vi "Simulation DIP.vi"() -> ()   [LabVIEW 2014]
uses:
  <vilib>/Simulation/Scripting/Companion Diagram/SimConfigNode/SimParams.ctl
  <vilib>/Simulation/Scripting/Companion Diagram/SimConfigNode/_simSolvers.ctl
  <vilib>/Simulation/Implementation/Shared/SIMSCR Execution Mode.ctl
  <vilib>/Simulation/Param Hierarchy/Typedefs/SIMPH Param Control Actions.ctl
  <vilib>/Simulation/Implementation/Shared/NILVSim_ParamChanged.vi
  <vilib>/Simulation/Implementation/Shared/NILVSIM_BeginStep.vi
  <vilib>/Simulation/Utility/Implementation/SIM Halt.vi
  <vilib>/Simulation/SignalArithmetic/Implementation/NILVSim Gain.llb/SIM Gain (scalar).vi
  <vilib>/Simulation/Implementation/Shared/SIM Is Init or Final Stage.vi
  <vilib>/Simulation/ContinuousLinear/Implementation/NILVSim State Space.llb/SIM State Space Distributor (SISO CD).vi
  <vilib>/Simulation/SignalArithmetic/Implementation/NILVSim Gain.llb/SIM Gain (vector,MatrixGain).vi
  <vilib>/Simulation/ContinuousLinear/Implementation/NILVSim State Space.llb/SIM State Space Collector (SISO CD).vi
  <vilib>/Simulation/SignalArithmetic/Implementation/NILVSim Gain.llb/SIM Gain (vector).vi
  <vilib>/Simulation/Implementation/Shared/NILVSim_Manager.vi
  <vilib>/Utility/error.llb/Clear Errors.vi
  <vilib>/Simulation/Implementation/Shared/NILVSim_FinalizeModel.vi
  <vilib>/addons/Control Design/_Model Construction/Model Creation.llb/Model Creation SubVI/cd_Create State Space Model.vi
  <vilib>/addons/Control Design/_Utility/Model Viewer.llb/Model Viewer SubVI/cd_Draw State-Space Equation (SS).vi
  <vilib>/addons/Control Design/_State Feedback Control/State Feedback Control.llb/State Feedback Control SubVis/cd_Linear Quadratic Regulator.vi
  <vilib>/Simulation/Implementation/Shared/SIM Unbundle Sim Info.vi
  <vilib>/Simulation/Implementation/Shared/NILVSim_Initialize.vi
  <vilib>/Simulation/Utility/Implementation/NILVSim Get Time and IsAcceptedStep.vi
  <vilib>/Simulation/Implementation/Shared/SIMSH Read Queue.vi
  <vilib>/Simulation/Implementation/Shared/NILVSim_GetModelError.vi
  <vilib>/Simulation/Implementation/Shared/SIM Bundle Sim Info.vi
  <vilib>/Simulation/Scripting/Companion Diagram/SimConfigNode/SimDog.xnode
  NL-Modell-Doppelpendel.vi
  <vilib>/addons/Control Design/_Model Construction/Model Typedefs.llb/CD State Space Model (MIMO).ctl
  <vilib>/addons/Control Design/_Model Construction/Model Typedefs.llb/CD General Elements.ctl
  <vilib>/Simulation/Implementation/XNodeFramework/SimXNode/SimX.xnode
  <vilib>/addons/Control Design/_Model Construction/NI_LinSys_Model Typedefs.lvlib
  <vilib>/addons/Control Design/_State Feedback Control/NI_CD_State Feedback Control.lvlib
  <vilib>/addons/Control Design/_Utility/NI_CD_Model Viewer.lvlib
  <vilib>/addons/Control Design/_Model Construction/NI_LinSys_Model Creation.lvlib
  <vilib>/Simulation/ContinuousLinear/Implementation/NILVSim State Space.llb/SIM State Space (SISO CD).vi
  <vilib>/Simulation/Implementation/Shared/NI_SIM_Implementation.lvlib
panel:
  in  "n":dbl
  out "E p 2":cluster{" 4":sgl, " 4":sgl, " 4":sgl}(graph)
  out "E p":sgl(graph)
  out "E t":dbl(graph)
  in  "ke":dbl
  in  "kv":dbl
  in  "kx":dbl
  in  "Regler 2":bool
  out "Winkel 2(Grad)":dbl(graph)=-0.008492510240475513
  out "Winkelgeschwindigkeit 2":cluster{dbl, "x4_":dbl}(graph)={5.3984229717087e-05, "x4_"=5.3984229717087e-05}
  in  "Regler":enum16{"kein", "PBR", "LQR"}(ring)=enum."LQR"
  in  "Winkelg.2_t0":dbl
  in  "Winkel2_t0 (Grad)":dbl
  in  "Winkelg.1_t0":dbl
  in  "Position_t0 (m)":dbl
  out "Kraft in N":dbl=-0.0022267318727753616
  out "Winkelgesch. Simuliert":dbl=1.2061069581493266e-05
  out "Winkel1  (rad)":dbl=-2.7704816976115154e-05
  out "Geschwindigkeit 2":dbl=0.00013263924275168403
  out "Position":dbl=0.9161585295653075
  in  "Strecke":T1(ring)
  out "State-Space Equation":picture
  out "Position (mm)":cluster{"output":dbl, "output":dbl}(graph)={"output"=100.0, "output"=0.9161585295653075}
  out "Winkel 1(Grad)":dbl(graph)=-0.001587369084913794
  out "Kraft (N)":dbl(graph)=-0.0022267318727753616
  out "Geschwindigkeit":dbl(graph)=0.00013263924275168403
  out "Winkelgeschwindigkeit 1":cluster{dbl, "x4_":dbl}(graph)={1.2061069581493266e-05, "x4_"=1.2061069581493266e-05}
  out "K":dbl[][](array[numeric])=[[99.99999999995181, -969.5856366468216, 394.3194914179953, 252.01094744906607, 27.114441675359792, 156.37982209545834]] format="%.2f"
  in  "Q":dbl[][](array[numeric])=[[100.0, 0.0, 0.0, 0.0, 0.0, 0.0], [0.0, 1.0, 0.0, 0.0, 0.0, 0.0], [0.0, 0.0, 100.0, 0.0, 0.0, 0.0], [0.0, 0.0, 0.0, 1.0, 0.0, 0.0], [0.0, 0.0, 0.0, 0.0, 1.0, 0.0], [0.0, 0.0, 0.0, 0.0, 0.0, 1.0]] format="%.2f"
  in  "R":dbl[][](array[numeric])=[[0.01]] format="%.5f"
  in  "Winkel1_t0 (Grad)":dbl
  in  "Sollwert Amplitude (mm)":dbl=100.0
  in  "Stop Button":bool
  # "Anfangswerte"
  # "PBR"
  # "LQR Regler"
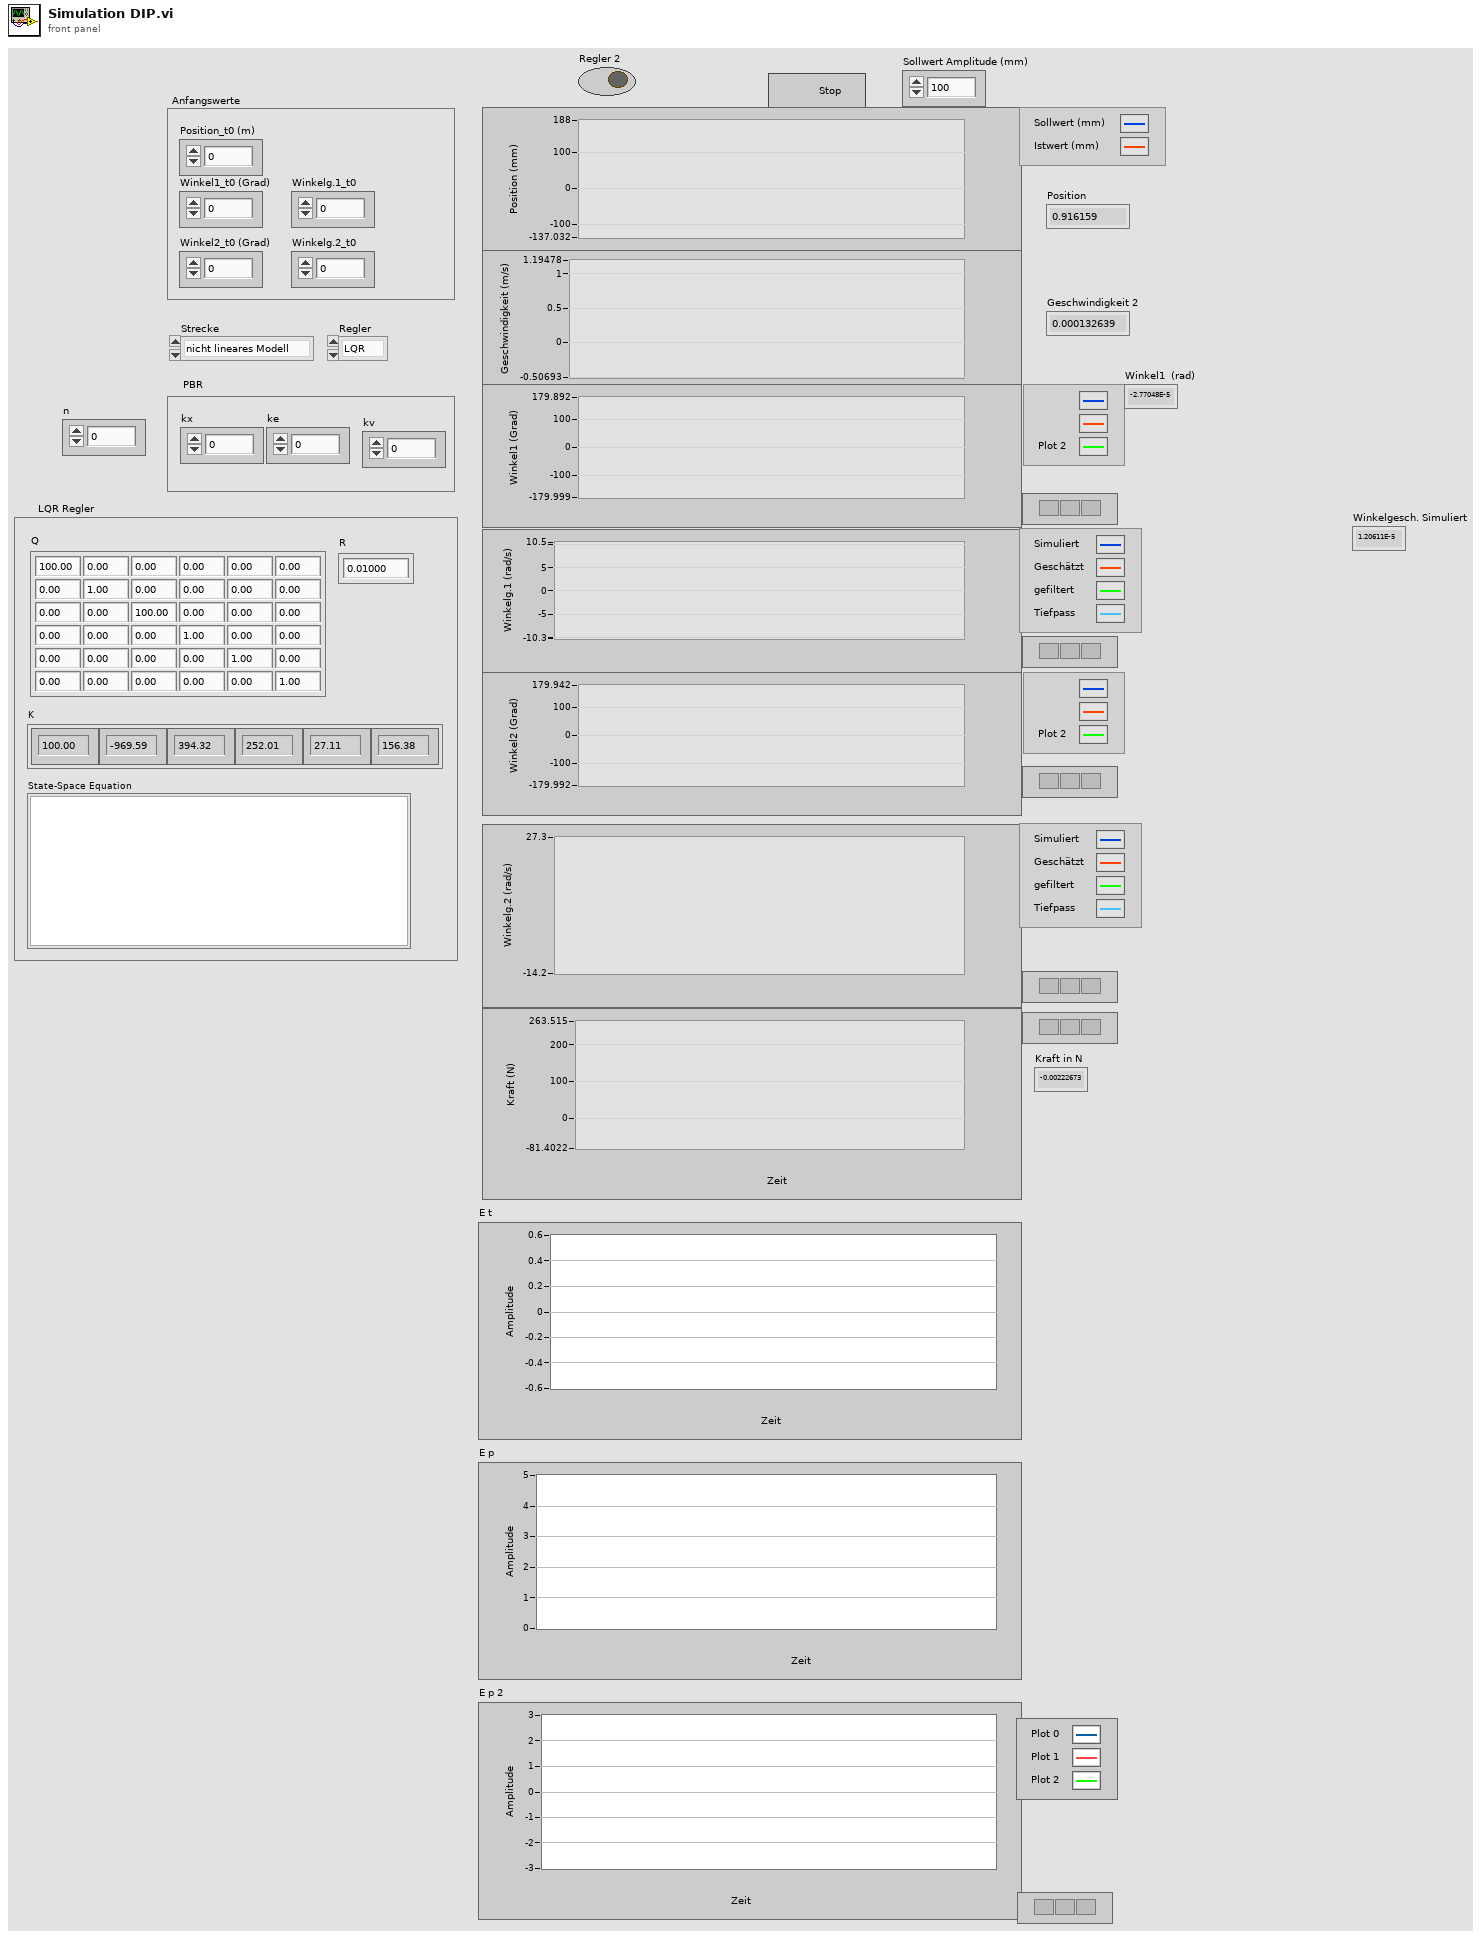
[diagram p1: front panel]
types:
  T1 = enum16{"nicht lineares Modell", "lineares Modell"}
  T2 = typedef "NI_LinSys_Model Typedefs.lvlib/CD State Space Model (MIMO).ctl" = cluster{"properties":T3, "A":dbl[][], "B":dbl[][], "C":dbl[][], "D":dbl[][], "StateNames":string[], "Transport Delay":dbl[][]}
  T3 = typedef "NI_LinSys_Model Typedefs.lvlib/CD General Elements.ctl" = cluster{"Model name":string, "Input names":string[], "Output names":string[], "Input Delays":dbl[], "Output Delays":dbl[], "Sampling Time":dbl, "Notes":string}
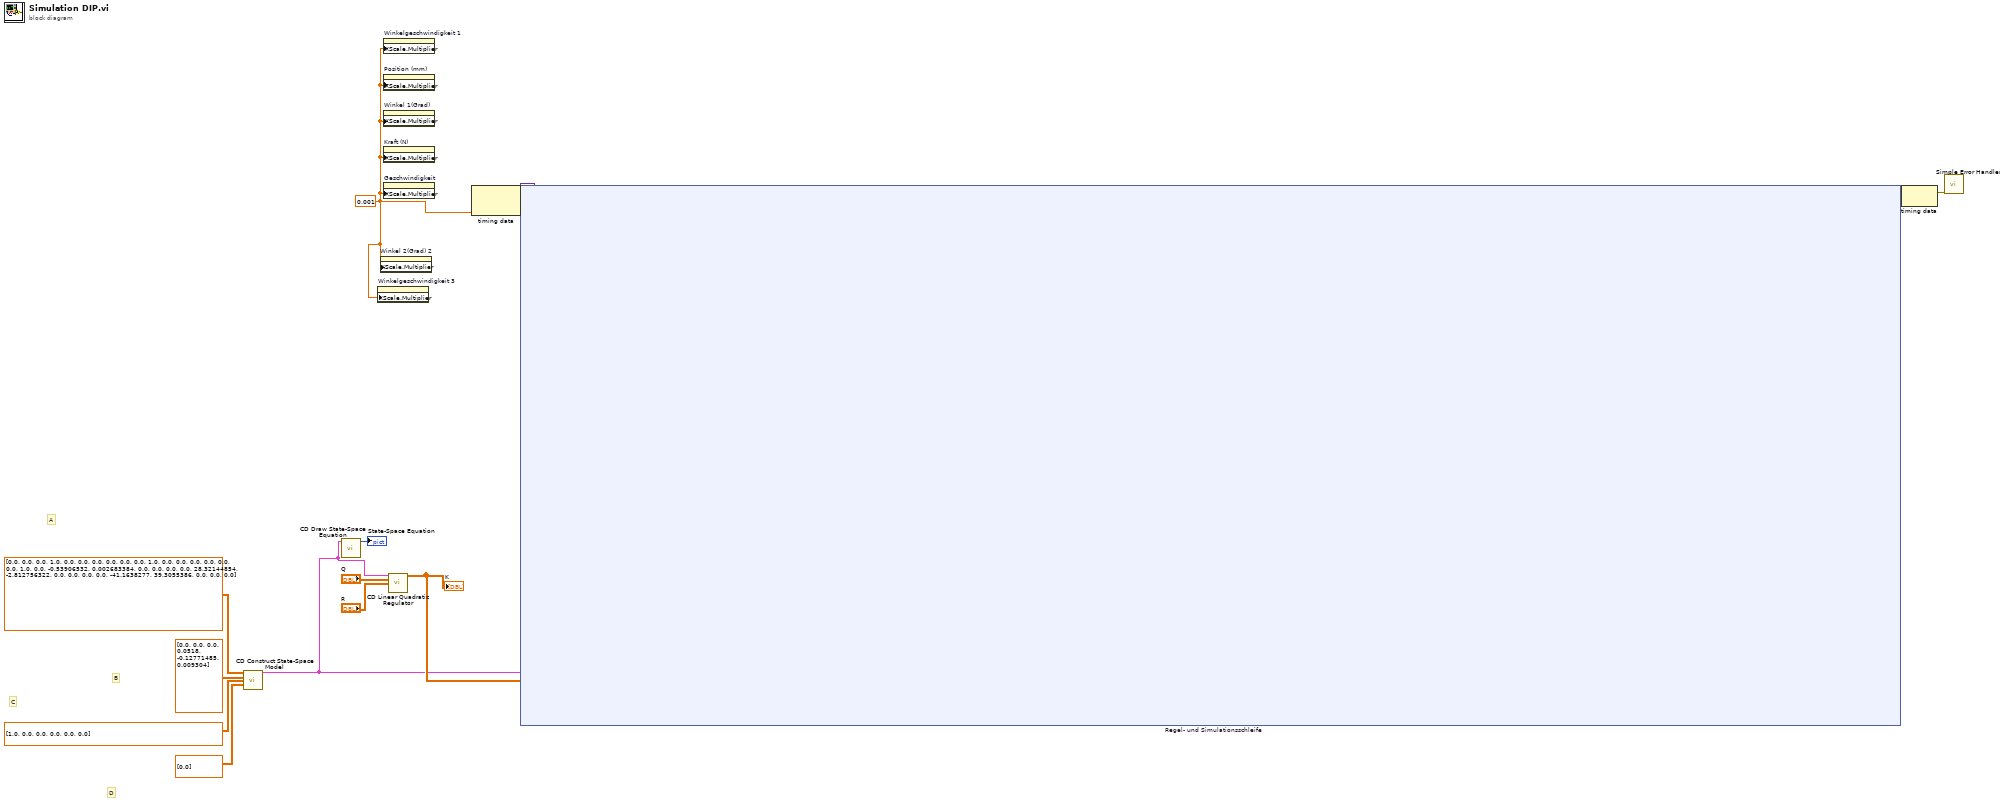
[diagram p0: block diagram]
diagram:
  w6 = 0.001 ("Step Size (s)")
  # "D"
  # "C"
  # "B"
  # "A"
  n1 = call-poly <vilib>:"CD Construct State-Space Model.vi"("A"=dbl[][] [[0.0, 0.0, 0.0, 1.0, 0.0, 0.0], [0.0, 0.0, 0.0, 0.0, 1.0, 0.0], [0.0, 0.0, 0.0, 0.0, 0.0, 1.0], [0.0, -0.53906532, 0.002683384, 0.0, 0.0, 0.0], [0.0, 28.32144854, -2.812756322, 0.0, 0.0, 0.0], [0.0, -41.1638277, 39.3055386, 0.0, 0.0, 0.0]], "B"=dbl[][] [[0.0], [0.0], [0.0], [0.0518], [-0.12771485], [0.009304]], "C"=dbl[][] [[1.0, 0.0, 0.0, 0.0, 0.0, 0.0]], "D"=dbl[][] [[0.0]]) -> ("State-Space Model"=w1:T2)  [unwired: 10 in, 1 out]
  n2 = call-poly <vilib>:"CD Draw State-Space Equation.vi"("State-Space Model"=w1) -> ("Equation"=→"State-Space Equation":picture)  [unwired: 8 in, 2 out]
  n3 = property on="Winkelgeschwindigkeit 3" class="SVDiagr (strikt)"("XScale.Multiplier"=w6) -> ()  [unwired: 2 in, 2 out]
  n4 = property on="Winkel 2(Grad) 2" class="SVDiagr (strikt)"("XScale.Multiplier"=w6) -> ()  [unwired: 2 in, 2 out]
  n5 = property on="Winkelgeschwindigkeit 1" class="SVDiagr (strikt)"("XScale.Multiplier"=w6) -> ()  [unwired: 2 in, 2 out]
  n6 = property on="Position (mm)" class="SVDiagr (strikt)"("XScale.Multiplier"=w6) -> ()  [unwired: 2 in, 2 out]
  n7 = property on="Winkel 1(Grad)" class="SVDiagr (strikt)"("XScale.Multiplier"=w6) -> ()  [unwired: 2 in, 2 out]
  n8 = property on="Kraft (N)" class="SVDiagr (strikt)"("XScale.Multiplier"=w6) -> ()  [unwired: 2 in, 2 out]
  n9 = property on="Geschwindigkeit" class="SVDiagr (strikt)"("XScale.Multiplier"=w6) -> ()  [unwired: 2 in, 2 out]
  n10 = call-poly <vilib>:"CD Linear Quadratic Regulator.vi"("State-Space Model"=w1, "Q"="Q", "R"="R") -> ("Optimal Gain (K)"=w2:dbl[][])  [unwired: 9 in, 3 out]
  "K" <- w2
  n11 = node-c288(w6) -> (w9:variant)  [unwired: 1 in]
  n12 = node-c254 "Regel- und Simulationsschleife"(w9, w1, w2) -> (w8:variant)
  n13 = node-c288(w8) -> (w7:errorcluster)
  n14 = call <vilib>:"Simple Error Handler.vi"("error in (no error)"=w7) -> ()  [unwired: 4 in, 5 out]
